vi "ID.vi"(8 "error in (no error)":errorcluster, 11 "Sensor in":refnum<class "Sensor Config.lvclass">) -> (0 "error out":errorcluster, 2 "ID":string, 3 "Sensor out":refnum<class "Sensor Config.lvclass">)   [LabVIEW 2020, in "VolatusConfig.lvlib" / "Sensor Config.lvclass"]
uses:
  Sensor Config.lvclass
  C:/dev/lv20CE/relink/lv-volatus/VolatusConfig/VolatusConfigElement/VolatusConfigElement.lvclass
  VolatusConfigElement/VolatusConfigElement.lvclass/VolatusConfigElement.ctl
  VolatusConfigElement/Element.vi
  Sensor Config.lvclass/Sensor Config.ctl
  VolatusConfigElement/VolatusConfigElement.lvclass
  lv-cdm/CDM-Config/Config Element/Config Element.lvclass
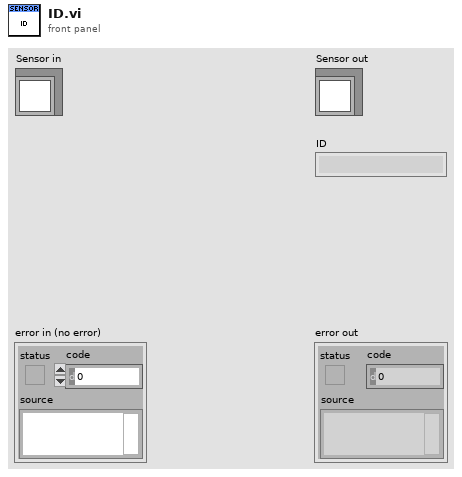
[diagram p1: front panel]
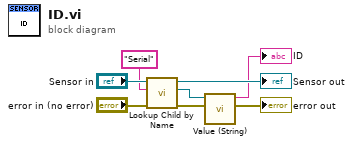
[diagram p0: block diagram]
diagram:
  n1 = call "Lookup Child by Name.vi"("error in (no error)"="error in (no error)", "Child Name"="Serial", "VolatusConfigElement in"="Sensor in") -> ("error out"=w4:errorcluster, "Child"=w3:refnum<class "Config Element.lvclass">, "VolatusConfigElement out"=→"Sensor out":refnum<class "Sensor Config.lvclass">)  [unwired: 5 in, 1 out]
  n2 = call "Value (String).vi"("error in (no error)"=w4, "Config Element in"=w3) -> ("error out"=→"error out":errorcluster, "String Value"=→"ID":string)  [unwired: 8 in]
